vi "ADS Load Classes.vi"(8 "error in (no error)":errorcluster, 10 "ref in":u64, 11 "Class name path":path) -> (0 "error out":errorcluster, 3 "ref out":u64)   [LabVIEW 2024]
uses:
  dependencies_dll_release/TCV_Lib.dll
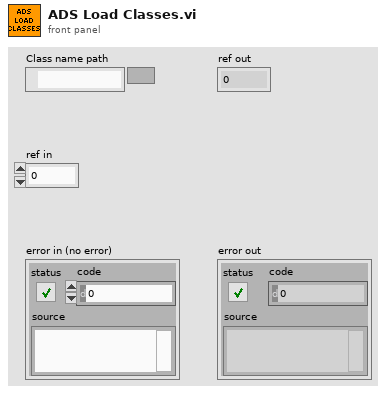
[diagram p1: front panel]
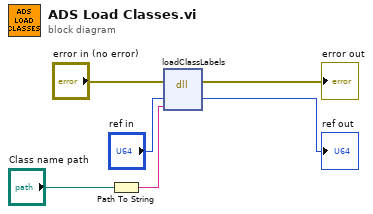
[diagram p0: block diagram]
diagram:
  n1 = Path To String(path="Class name path") -> (string=w2:string)
  n2 = dll-call lib="D:/labviewTestTCVdll/TransformCV-LabVIEW/Test/dependencies_dll_release/TCV_Lib.dll" fn="loadClassLabels"(error in="error in (no error)", "ref"="ref in", "class_names"=w2) -> (error out=→"error out":errorcluster, "ref"=→"ref out":u64)  [unwired: 4 in, 1 out]
